vi "get_context.vi"(8 "error in (no error)":errorcluster, 11 "Queue Log Provider in":refnum<class "Queue Log Provider.lvclass">) -> (0 "error out":errorcluster, 1 "context":string, 3 "Queue Log Provider out":refnum<class "Queue Log Provider.lvclass">)   [LabVIEW 2019, in "Queue Log Provider.lvclass"]
uses:
  Queue Log Provider.lvclass
  Queue Log Provider.lvclass/Queue Log Provider.ctl
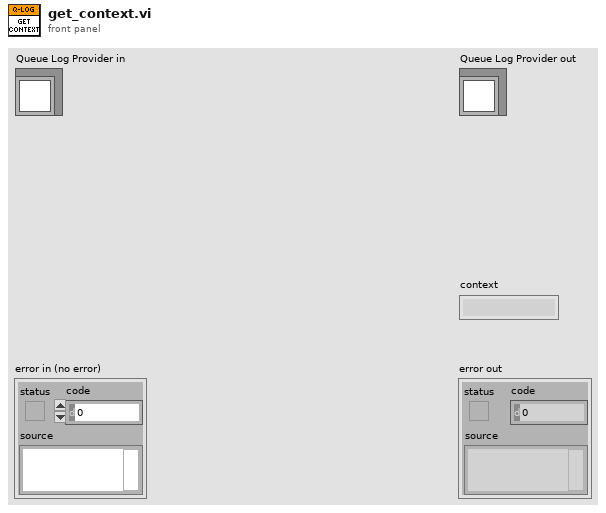
[diagram p1: front panel]
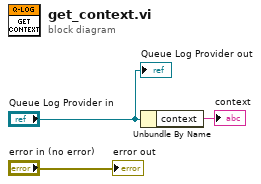
[diagram p0: block diagram]
diagram:
  n1 = Unbundle By Name("Queue Log Provider in") -> ("context"=→"context":string)
  "error out" <- "error in (no error)"
  "Queue Log Provider out" <- "Queue Log Provider in"
